vi "Log_Data.vi"(0 "File_Path_In":path, 5 "Input_Size (in kb)":i64, 11 "Error_In":errorcluster) -> (4 "File_Path_Out":path, 15 "Error_Out":errorcluster)   [LabVIEW 2023]
doc: "This VI logs the data that are generated to text file."
uses:
  Controls/Operation_Select_Queue.ctl
  <vilib>/regexp/Match Regular Expression.xnode
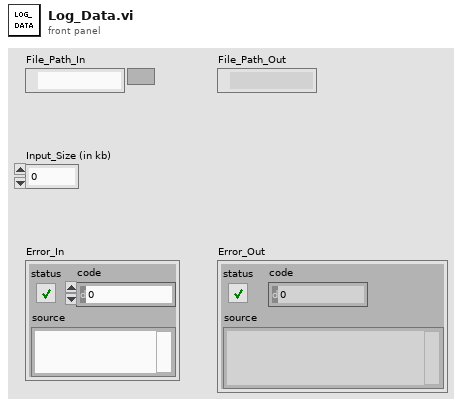
[diagram p1: front panel]
types:
  T1 = typedef "Operation_Select_Queue.ctl" = enum16{"Initialize", "Enqueue", "Dequeue", "Preview"}
  T2 = enum16{"open", "replace", "create", "open or create", "replace or create", "replace or create with confirmation"}
  T3 = typedef "Data.ctl" = cluster{"Generated_Data":dbl, "Time_Stamp":string}
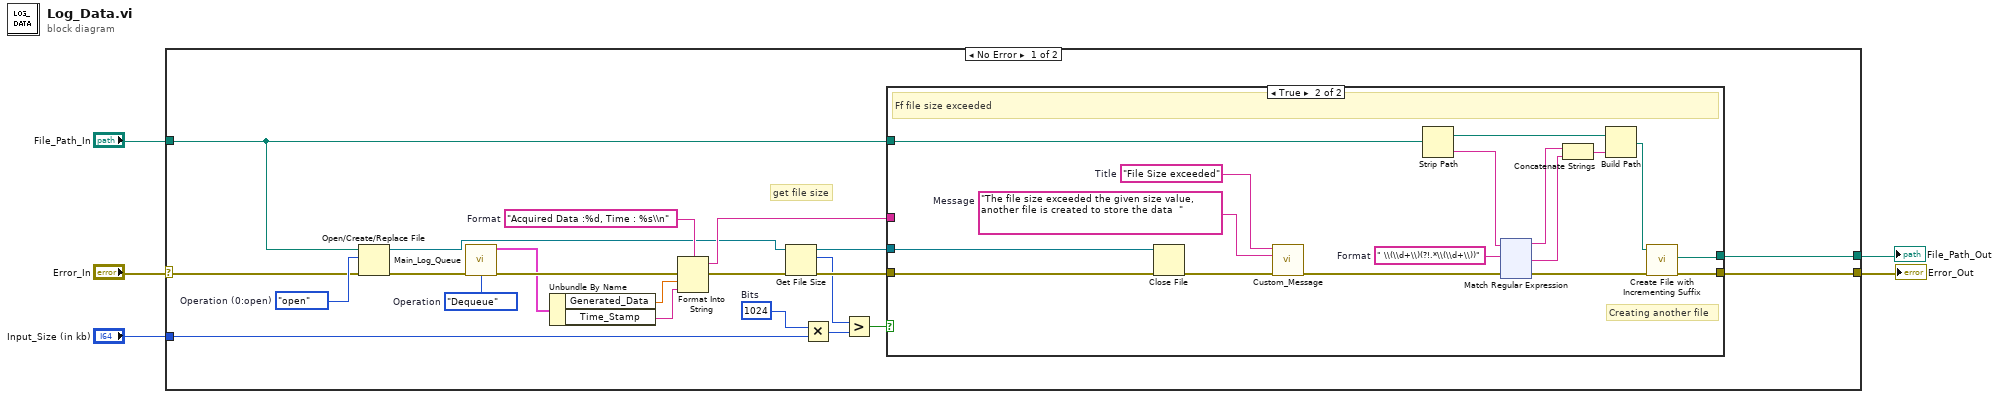
[diagram p0: block diagram]
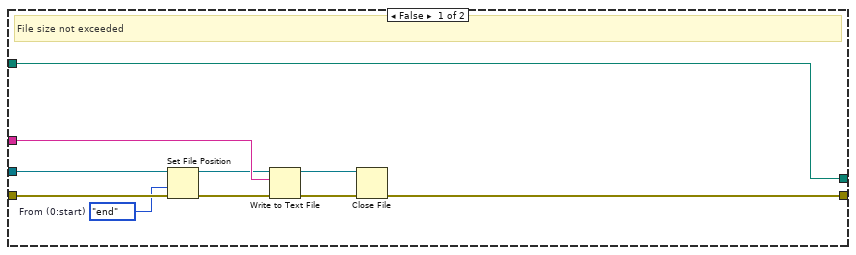
[diagram p2: hidden frame]
diagram:
  n1 = case shown="No Error" "Error_In" {
    selector: "Error_In" -> [w19 w173]
    tunnel: "File_Path_In" -> [w12 w172]
    tunnel: [w11 w173] -> w5
    tunnel: "Input_Size (in kb)" -> [w7 _]
    tunnel: [w10 w172] -> w2
    frame No Error {
      w6 = i64 1024  # Bits
      w20 = "Acquired Data :%d, Time : %s\\n"  # Format
      w25 = Operation_Select_Queue."Dequeue"  # Operation
      w27 = T2."open"  # Operation (0:open)
      # "get file size"
      n2 = Open/Create/Replace File(file path (use dialog)=w12, error in=w19, operation (0:open)=w27) -> (refnum out=w9:refnum<file>, error out=w26:errorcluster)  [unwired: 3 in, 1 out]
      n3 = call "Main_Log_Queue.vi"("Error_In"=w26, "Operation"=w25) -> ("Generated_Data_Out"=w23:T3, "Error_Out"=w24:errorcluster)  [unwired: 9 in, 3 out]
      n4 = Unbundle By Name(w23) -> ("Generated_Data"=w22:dbl, "Time_Stamp"=w21:string)
      n5 = Format Into String(format string=w20, error in=w24, w22, w21) -> (resulting string=w13:string, error out=w18:errorcluster)  [unwired: 1 in]
      n6 = Get File Size(file=w9, error in=w18) -> (refnum out=w16:refnum<file>, size (in bytes)=w14:i64, 0:w17:errorcluster)
      n7 = Multiply(x=w6, y=w7) -> (x*y=w8:i64)
      n8 = Greater?(x=w14, y=w8) -> (0:w15:bool)
      n9 = case shown="True" w15 {
        tunnel: [w35 w52] -> w11
        tunnel: w17 -> [w32 w51]
        tunnel: w16 -> [w31 w49]
        tunnel: w13 -> [w37 _]
        tunnel: w12 -> [w33 w47]
        tunnel: [w33 w48] -> w10
        frame False {
          w28 = enum16{"start", "end", "current"}."end"  # From (0:start)
          # "File size not exceeded"
          n10 = Set File Position(refnum=w31, from (0:start)=w28, error in=w32) -> (refnum out=w30:refnum<file>, error out=w29:errorcluster)  [unwired: 1 in]
          n11 = Write to Text File(file (use dialog)=w30, text=w37, error in=w29) -> (refnum out=w34:refnum<file>, error out=w36:errorcluster)  [unwired: 1 in, 1 out]
          n12 = Close File(refnum=w34, error in=w36) -> (error out=w35:errorcluster)  [unwired: 1 out]
        }
        frame True {
          w43 = " \\(\\d+\\)(?!.*\\(\\d+\\))"  # Format
          w53 = "File Size exceeded"  # Title
          w54 = "The file size exceeded the given size value, another file is created to store the data  "  # Message
          # "Creating another file"
          # "Ff file size exceeded"
          n13 = Close File(refnum=w49, error in=w51) -> (error out=w50:errorcluster)  [unwired: 1 out]
          n14 = call "Custom_Message.vi"("Title"=w53, "Message"=w54, "Error_In"=w50) -> ("Error_Out"=w39:errorcluster)  [unwired: 11 in, 1 out]
          n15 = Strip Path(path=w47) -> (stripped path=w45:path, name=w44:string)
          n16 = xnode "Match Regular Expression"("input string"=w44, "regular expression"=w43, "error in"=w39) -> ("before match"=w42:string, "after match"=w41:string, "error out"=w38:errorcluster)  [unwired: 3 in, 2 out]
          n17 = Concatenate Strings(w42, w41) -> (w40:string)
          n18 = Build Path(base path=w45, name or relative path=w40) -> (appended path=w46:path)
          n19 = call <vilib>:"Create File with Incrementing Suffix.vi"("error in (no error)"=w38, "file path"=w46) -> ("error out"=w52:errorcluster, "actual path"=w48:path)  [unwired: 7 in, 1 out]
        }
      }
    }
    frame Error {
    }
  }
  "Error_Out" <- w5
  "File_Path_Out" <- w2
